vi "Basic Main.vi"() -> ()   [LabVIEW 2011, in "LVH-Xbox-One-Controller.lvlib"]
uses:
  LVH-Xbox-One-Controller.lvlib
  Private/Type Defs/Indicators/A.ctl
  Private/Type Defs/Indicators/B.ctl
  Private/Type Defs/Indicators/X.ctl
  Private/Type Defs/Indicators/Y.ctl
  Async Worker.vi
  <vilib>/Utility/inputDevices.llb/closeJoystick.vi
panel:
  out "Y Button":T1 caption="Blank Button"
  out "X Button":T2 caption="Blank Button"
  out "B Button":T3 caption="Blank Button"
  out "A Button":T4 caption="Blank Button"
  in  "Stop Button":bool
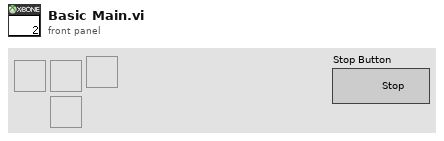
[diagram p1: front panel]
types:
  T1 = typedef "LVH-Xbox-One-Controller.lvlib/Y.ctl" = bool
  T2 = typedef "LVH-Xbox-One-Controller.lvlib/X.ctl" = bool
  T3 = typedef "LVH-Xbox-One-Controller.lvlib/B.ctl" = bool
  T4 = typedef "LVH-Xbox-One-Controller.lvlib/A.ctl" = bool
  T5 = cluster{"A":refnum<user-event>, "B":refnum<user-event>}
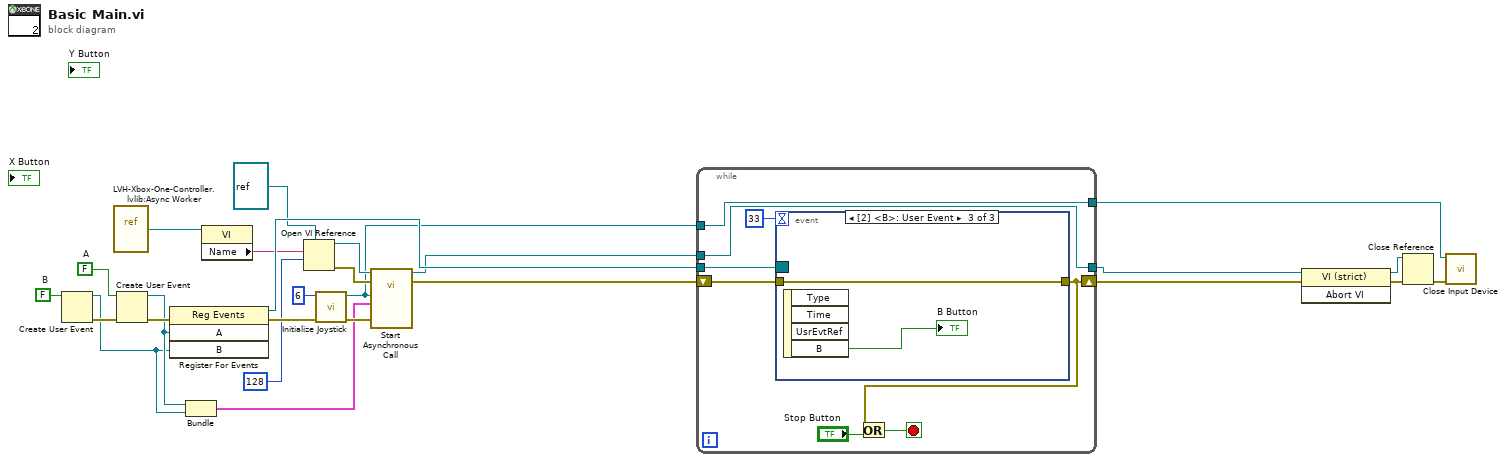
[diagram p0: block diagram]
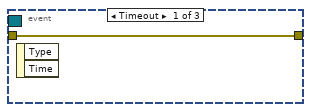
[diagram p2: hidden frame]
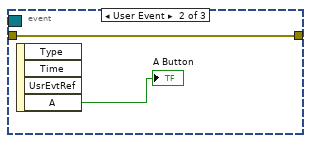
[diagram p3: hidden frame]
diagram:
  w25 = FALSE  # B
  w26 = FALSE  # A
  n1 = Create User Event(user event datatype=w25) -> (user event=w19:refnum<user-event>, error out=w24:errorcluster)  [unwired: 1 in]
  n2 = vi-ref "LVH-Xbox-One-Controller.lvlib:Async Worker.vi"() -> (w17:refnum<vi>)
  n3 = Create User Event(user event datatype=w26, error in=w24) -> (user event=w20:refnum<user-event>, error out=w23:errorcluster)
  n4 = register-events(error in=w23, w20, w19) -> (reference out=w22:refnum<event-registration>, error out=w18:errorcluster)  [unwired: 1 in]
  n5 = Bundle("A"=w20, "B"=w19) -> (w10:T5)  [unwired: 1 in]
  n6 = property class="VI"(reference=w17) -> ("Name"=w12:string)  [unwired: 1 in, 2 out]
  n7 = Open VI Reference(type specifier VI Refnum (for type only)=refnum<vi> refnum, vi path=w12, options=128) -> (vi reference=w14:refnum<vi>, error out=w13:errorcluster)  [unwired: 3 in]
  n8 = call <vilib>:"Initialize Joystick.vi"("error in (no error)"=w18, "device index"=6) -> ("error out"=w11:errorcluster, "device ID"=w1:refnum<k1>)  [unwired: 8 in]
  n9 = call-by-ref "Start Asynchronous Call"(reference=w14, error in=w13, 8:"error in (no error)"=w11, "Events"=w10, "Controller Ref"=w1) -> (reference out=w9:refnum<vi>, error out=w8:errorcluster)  [unwired: 6 in, 3 out]
  n10 = while {
    tunnel: w22 -> [w34]
    shift-right: [w27] -> w4
    shift-left: w8 -> [w30]
    tunnel: w9 -> [w29]
    tunnel: [w29] -> w5
    tunnel: [w28] -> w2
    tunnel: w1 -> [w28]
    stop <- w31 stop-if-true
    n11 = event shown="[2] <B>: User Event" {
      selector: w34 -> [_ _ _]
      dyn-events: _ -> [_ _ _]
      timeout: 33 -> [_ _ _]
      tunnel: w30 -> [w35 w37 w39]
      tunnel: [w35 w37 w39] -> w27
      event Timeout {
        n12 = event-data() -> ()  [unwired: 1 in, 2 out]
      }
      event User Event {
        n13 = event-data() -> ("A"=→"A Button":bool)  [unwired: 1 in, 3 out]
      }
      event User Event {
        n14 = event-data() -> ("B"=→"B Button":bool)  [unwired: 1 in, 3 out]
      }
    }
    n15 = Or(x=w27, y="Stop Button") -> (x .or. y?=w31:bool)
  }
  n16 = invoke class="VI (strict)" method="Abort VI"(reference=w5, error in=w4) -> (reference out=w6:refnum<vi>, error out=w7:errorcluster)  [unwired: 1 in, 1 out]
  n17 = Close Reference(reference=w6, error in (no error)=w7) -> (error out=w3:errorcluster)
  n18 = call-poly <vilib>:"Close Input Device.vi"("error in (no error)"=w3, "device ID"=w2) -> ()  [unwired: 8 in, 1 out]
